vi "Entry.vi"(8 "error in (no error)":errorcluster, 11 "New State":refnum<class "Localize.lvclass">) -> (0 "error out":errorcluster, 3 "State out":refnum<class "Localize.lvclass">)   [LabVIEW 2014, in "States.lvlib" / "Localize.lvclass"]
doc: "This is an abstract method. Override this method to define the behavior when you enter the state."
uses:
  Localize.lvclass
  <vilib>/ActorFramework/Message Enqueuer/Message Enqueuer.lvclass/Message Enqueuer.ctl
  <vilib>/ActorFramework/Message Enqueuer/Enqueue.vi
  <vilib>/ActorFramework/Message Priority Queue/Priority Enqueue.vi
  Process State/CoordinatorState.lvclass
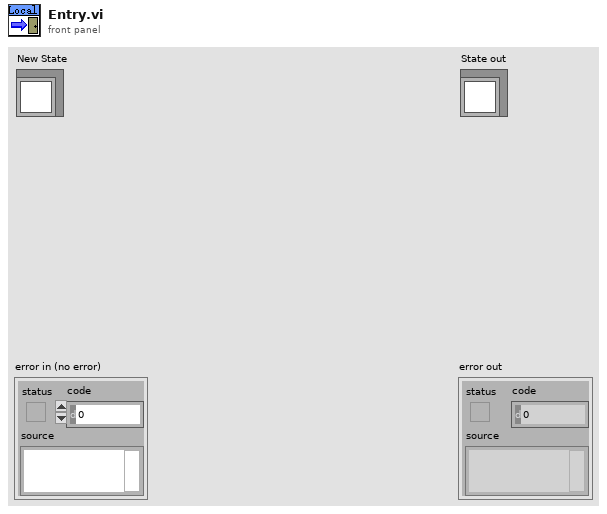
[diagram p1: front panel]
types:
  T1 = enum32{"Joy", "Map", "Voice", "Input", "Undefined"}
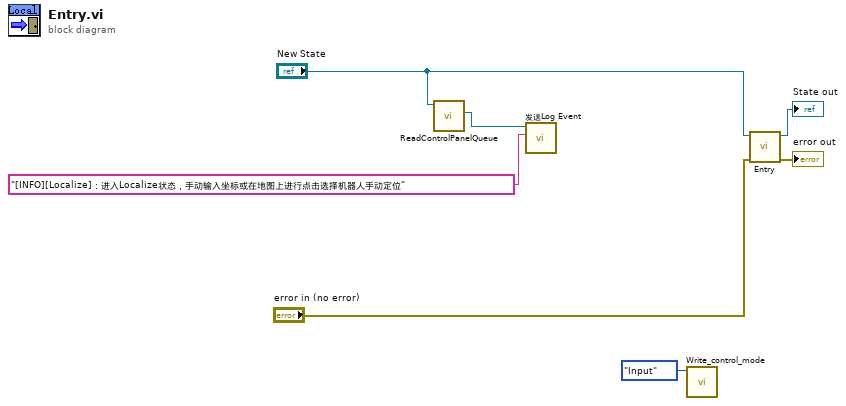
[diagram p0: block diagram]
diagram:
  n1 = call-dynamic "ReadControlPanelQueue.vi"("CoordinatorState输入"="New State") -> ("操作者框架:消息待入队列"=w2:refnum<class "Message Enqueuer.lvclass">)  [unwired: 8 in, 2 out]
  n2 = call "发送Log Event.vi"("Event Text"="[INFO][Localize]：进入Localize状态，手动输入坐标或在地图上进行点击选择机器人手动定位", "消息待入队列"=w2) -> ()  [unwired: 8 in, 2 out]
  n3 = call "Write_control_mode.vi"("Control_Mode"=T1."Input") -> ()  [unwired: 11 in]
  n4 = call-parent "Entry.vi"("error in (no error)"="error in (no error)", "New State"="New State") -> ("error out"=→"error out":errorcluster, "State out"=→"State out":refnum<class "Localize.lvclass">)  [unwired: 8 in]
